vi "队列初始化.vi"() -> (3 "输出队列":T1)   [LabVIEW 2014]
uses:
  Controls/Cam1QueueAction.ctl
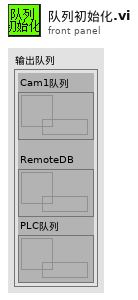
[diagram p1: front panel]
types:
  T1 = cluster{"Cam1队列":refnum<queue>, "RemoteDB":refnum<queue>, "PLC队列":refnum<queue>}
  T2 = typedef "欧姆龙PLC Action.ctl" = enum16{"读设备状态", "初始化", "待命", "重新初始化", "读触发信息", "读第1组Mark点坐标", "读第2组Mark点坐标", "写基本信息", "写第1组Mark点坐标", "写第2组Mark点坐标", "写相机中心到出线头的距离", "写一笔轨迹到PLC", "写入进线前段点位", "写入板内布线点位", "写入出线布线点位", "写入数据写入完成信号", "获取信息", "写入进出线方向", "写加工信号"}
  T3 = typedef "Cam1QueueAction.ctl" = enum16{"Cam1初始化", "Cam1更新曝光时间-拍Mark点1", "Cam1更新曝光时间-拍Mark点2", "Cam1更新曝光时间-拍照二维码", "Cam1待命", "Cam1实时-Mark", "Cam1实时-二维码", "Cam1手动:Mark1", "Cam1手动:Mark2", "Cam1手动:二维码", "Cam1自动:Mark1", "Cam1自动:Mark2"}
  T4 = cluster{"queue out":refnum<queue>, "queue out":refnum<queue>, "queue out":refnum<queue>}
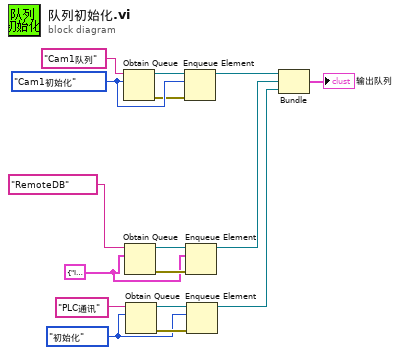
[diagram p0: block diagram]
diagram:
  w4 = cluster{"msg":string, "Data":variant} {"msg"="Initialize", "Data"=variant}
  w5 = 欧姆龙PLC_Action."初始化" ("欧姆龙PLC Action")
  w16 = Cam1QueueAction."Cam1初始化" ("PLC动作")
  n1 = Obtain Queue(name (unnamed)="Cam1队列" ("名称（未命名）"), element data type=w16) -> (queue out=w14:refnum<queue>, error out=w9:errorcluster)  [unwired: 3 in, 1 out]
  n2 = Obtain Queue(name (unnamed)="RemoteDB" ("名称（未命名）"), element data type=w4) -> (queue out=w12:refnum<queue>, error out=w10:errorcluster)  [unwired: 3 in, 1 out]
  n3 = Obtain Queue(name (unnamed)="PLC通讯" ("名称（未命名）"), element data type=w5) -> (queue out=w7:refnum<queue>, error out=w8:errorcluster)  [unwired: 3 in, 1 out]
  n4 = Enqueue Element(queue=w14, element=w16, error in (no error)=w9) -> (queue out=w13:refnum<queue>)  [unwired: 1 in, 2 out]
  n5 = Enqueue Element(queue=w12, element=w4, error in (no error)=w10) -> (queue out=w3:refnum<queue>)  [unwired: 1 in, 2 out]
  n6 = Enqueue Element(queue=w7, element=w5, error in (no error)=w8) -> (queue out=w2:refnum<queue>)  [unwired: 1 in, 2 out]
  n7 = Bundle("queue out"=w13, "queue out"=w3, "queue out"=w2) -> (→"输出队列":T4)  [unwired: 1 in]
